vi "ArraySimulation.vi"() -> ()   [LabVIEW 2013]
panel:
  in  "Smoothing":bool
  out "Sensor Frequencies (kHz)":dbl[](array[numeric])=[0.17730319811611386, 0.32537459895651155, 0.5187714918544717, 0.7567965602561179, 0.5935073569609096, 0.3847090964708457, 0.22207639875594293]
  out "Standardabweichung":dbl(slide)=nan scale=-1.0..9.023237115954172
  out "Einfallswinkel":dbl(knob) scale=-90.0..90.0
  in  "Gaussian Fit":bool
  in  "Stop Button":bool
  in  "Noise Strength":dbl
  in  "Lichteinfallswinkel":dbl(knob)=5.0142207518499475 scale=-90.0..90.0
  in  "Base Irradiance µW/cm²":dbl(knob)=0.9023237115954172 scale=0.001..1000.0
  # "Westen"
  # "Osten"
  # "Die Standardabweichung gilt über alle\nWerte und ist daher in dieser Form nur in der\nSimulation ein Maß für die Genauigkeit."
  # "Osten"
  # "Westen"
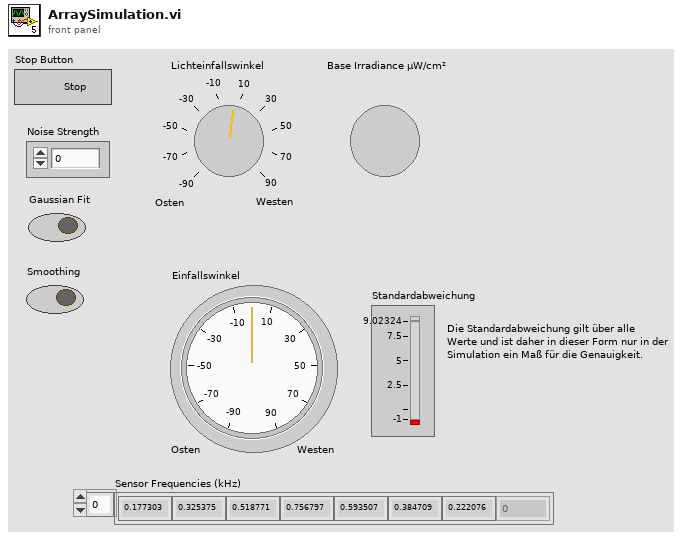
[diagram p1: front panel]
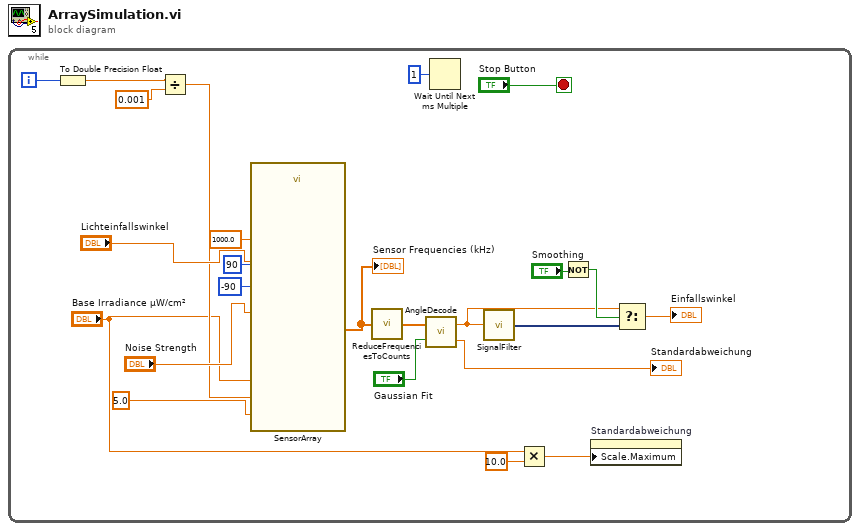
[diagram p0: block diagram]
diagram:
  n1 = while {
    i -> [w22]
    stop <- "Stop Button" stop-if-true
    n2 = To Double Precision Float(number=w22) -> (double precision float=w23:dbl)
    n3 = Divide(x=w23, y=0.001) -> (x/y=w14:dbl)
    n4 = call "SensorArray.vi"("Lichteinfallswinkel"="Lichteinfallswinkel", "Time s"=w14, "VDD V"=5.0, "Noise Strength"="Noise Strength", "Minimum Angle"=i8 -90, "Base Irradiance µW/cm²"="Base Irradiance µW/cm²", "Maximum Angle"=i8 90, "Gain"=1000.0) -> ("Sensor Frequencies (kHz)"=w13:dbl[])  [unwired: 5 in, 2 out]
    "Sensor Frequencies (kHz)" <- w13
    n5 = call "ReduceFrequenciesToCounts.vi"("Sensor Frequencies (kHz)"=w13) -> ("Sensor Counts"=w12:dbl[])
    n6 = call "AngleDecode.vi"("Interpolate"="Gaussian Fit", "Data"=w12) -> ("Standard Deviation"=→"Standardabweichung":dbl, "Peak Angle"=w5:dbl)
    n7 = Wait Until Next ms Multiple(millisecond multiple=u32 1) -> ()  [unwired: 1 out]
    n8 = call "SignalFilter.vi"("Signal In"=w5) -> ("Filtered Signal"=w8:dynamicdata)
    n9 = Multiply(x="Base Irradiance µW/cm²", y=10.0) -> (x*y=w3:dbl)
    n10 = Not(x="Smoothing") -> (.not. x?=w6:bool)
    n11 = property on="Standardabweichung" class="Slide (strict)"("Scale.Maximum"=w3) -> ()  [unwired: 2 in, 2 out]
    n12 = Select(t=w5, s=w6, f=w8) -> (s? t:f=→"Einfallswinkel":dbl)
  }
